vi "Get-action-default-settings.vi"(8 "error in (no error)":errorcluster, 9 "Motor actions":T1, 10 "Action in":refnum<class "Action.lvclass">, 11 "Motor in":refnum<class "Motor-Zaxis.lvclass">) -> (0 "error out":errorcluster, 2 "Action":refnum<class "Action.lvclass">, 3 "Motor out":refnum<class "Motor-Zaxis.lvclass">)   [LabVIEW 2013, in "PowderDeposition.lvlib" / "Motor-Zaxis.lvclass"]
uses:
  Motor-Zaxis.lvclass
  Action/Motor-actions.ctl
  Action/Action.lvclass
  Action/Move-Relative/Move-Relative.lvclass
  Action/Move-Relative/Move-Relative-settings.ctl
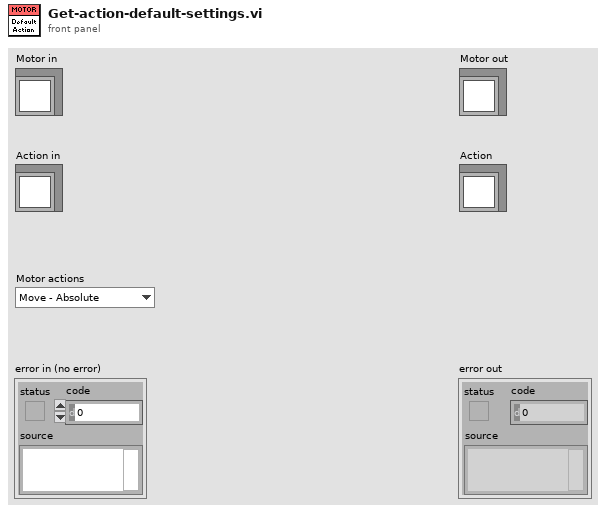
[diagram p1: front panel]
types:
  T1 = typedef "PowderDeposition.lvlib/Action.lvclass/Motor-actions.ctl" = enum16{"Move - Absolute", "Move - Relative", "Move - Timer", "Wait", "Home", "Substrate", "Sieve", "Stop"}
  T2 = typedef "PowderDeposition.lvlib/Move-Relative.lvclass/Move-Relative-settings.ctl" = cluster{"Displacement":dbl, "Speed":dbl, "Direction":enum16{"Clockwise", "Counter-clockwise"}, "Min duration":dbl}
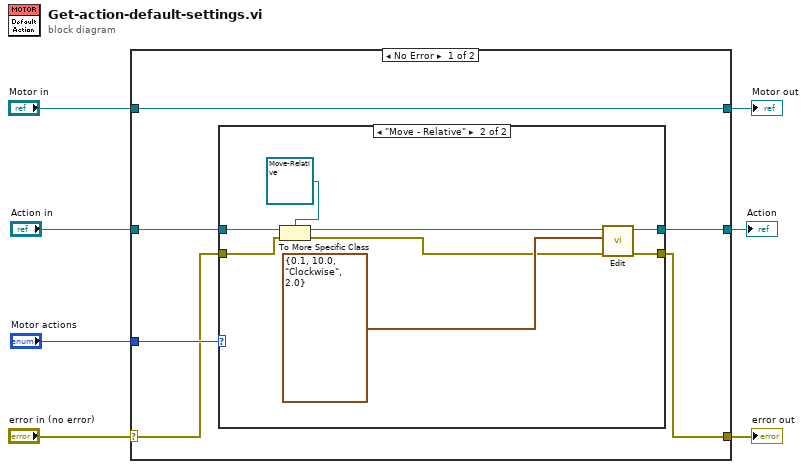
[diagram p0: block diagram]
diagram:
  n1 = case shown="No Error" "error in (no error)" {
    selector: "error in (no error)" -> [w9 w26]
    tunnel: [w8 w26] -> w6
    tunnel: [w13 w25] -> w4
    tunnel: "Motor in" -> [w13 w25]
    tunnel: "Motor actions" -> [w11 _]
    tunnel: "Action in" -> [w12 w24]
    tunnel: [w10 w24] -> w1
    frame No Error {
      n2 = case shown="\"Move - Relative\"" w11 {
        tunnel: w12 -> [w15 w23]
        tunnel: [w15 w20] -> w10
        tunnel: [w14 w17] -> w8
        tunnel: w9 -> [w14 w16]
        frame Default {
        }
        frame "Move - Relative" {
          n3 = To More Specific Class(target class=refnum<class "Move-Relative.lvclass"> refnum ("Move-Distance.lvclass"), reference=w23, error in=w16) -> (specific class reference=w21:refnum<class "Move-Relative.lvclass">, error out=w18:errorcluster)
          n4 = call-dynamic "Edit.vi"("error in (no error)"=w18, "Edit dialog"=T2 {"Displacement"=0.1, "Speed"=10.0, "Direction"=enum."Clockwise", "Min duration"=2.0}, "Action in"=w21) -> ("error out"=w17:errorcluster, "Action out"=w20:refnum<class "Move-Relative.lvclass">)  [unwired: 7 in]
        }
      }
    }
    frame Error {
    }
  }
  "error out" <- w6
  "Motor out" <- w4
  "Action" <- w1
